vi "GetVersion.vi"() -> ()   [LabVIEW 2013]
uses:
  <vilib>/Platform/fileVersionInfo.llb/FileVersionInformation.ctl
panel:
  out "FileVersionInfo Out":T1
  out "File Version Info":string
  in  "Visible":bool=TRUE
  in  "stop":bool
  in  "Version Message":string
  out "error out":errorcluster
  in  "error in (no error)":errorcluster
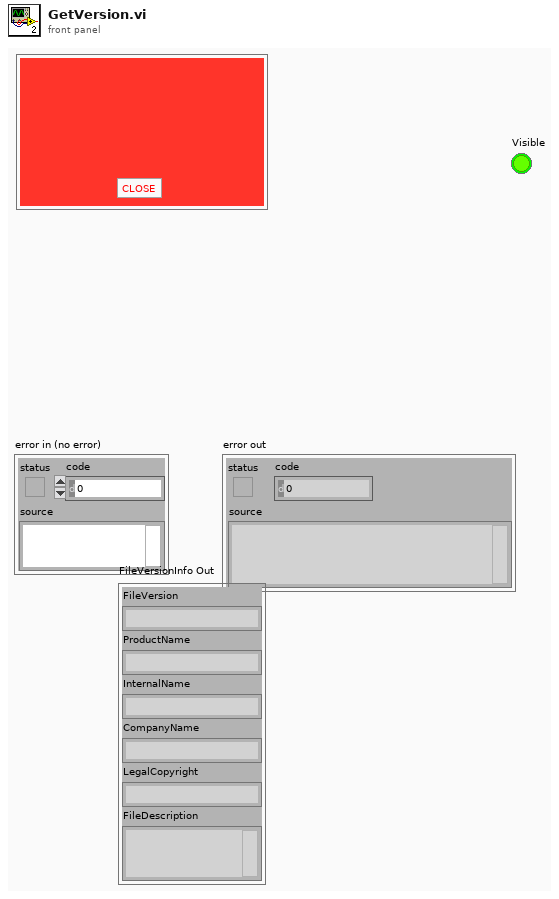
[diagram p1: front panel]
types:
  T1 = typedef "FileVersionInformation.ctl" = cluster{"FileVersion":string, "ProductName":string, "InternalName":string, "CompanyName":string, "LegalCopyright":string, "FileDescription":string}
  T2 = typedef "mysql_authentication.ctl" = cluster{"User":string, "Password":string, "Database":string}
  T3 = cluster{"Port":u16, "IP Address":string, "Authentication":T2}
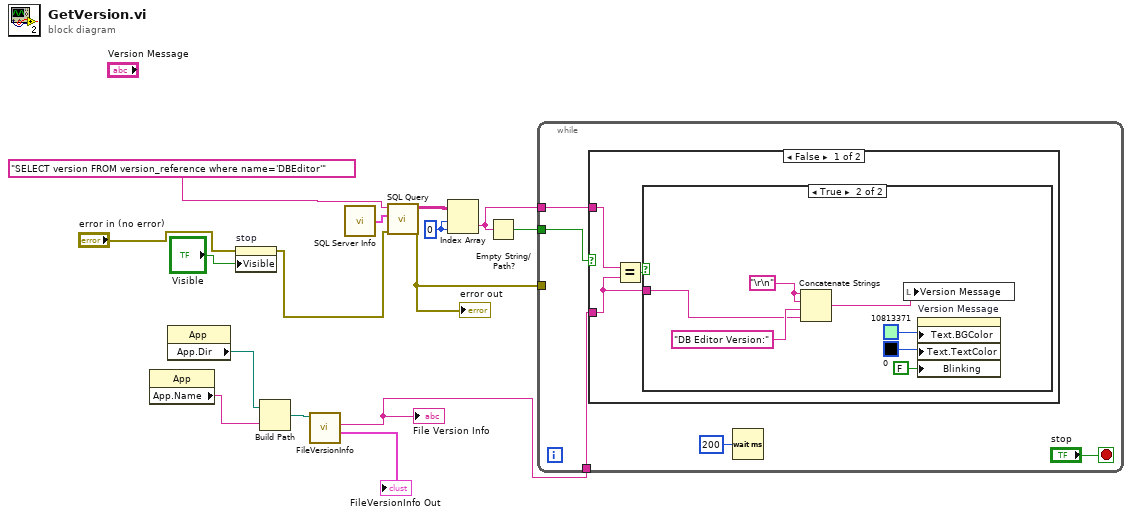
[diagram p0: block diagram]
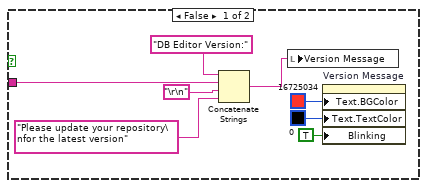
[diagram p2: hidden frame]
diagram:
  w12 = 0 ("disabled index (col)")
  n1 = property class="App"() -> ("App.Name"=w4:string)  [unwired: 2 in, 2 out]
  n2 = property class="App"() -> ("App.Dir"=w5:path)  [unwired: 2 in, 2 out]
  n3 = property on="stop" class="Bool"(error in="error in (no error)", "Visible"="Visible") -> (error out=w7:errorcluster)  [unwired: 1 in, 1 out]
  n4 = Build Path(base path=w5, name or relative path=w4) -> (appended path=w3:path)
  n5 = call <vilib>:"FileVersionInfo.vi"("Application Path in"=w3) -> ("FileVersionInfo Out"=→"FileVersionInfo Out":T1, "File Version Info"=w1:string)  [unwired: 7 in, 2 out]
  "File Version Info" <- w1
  n6 = call "SQL Server Info.vi"() -> ("SQL Server Info"=w14:T3)
  n7 = call "SQL Query.vi"("error in (no error)"=w7, "SQL Server Info"=w14, "Query"="SELECT version FROM version_reference where name='DBEditor'") -> ("error out"=w6:errorcluster, "data"=w15:string[][])  [unwired: 7 in]
  "error out" <- w6
  n8 = Index Array(array=w15, index (row)=w12, index (col)=w12) -> (element=w10:string)
  n9 = Empty String/Path?(string/path=w10) -> (empty?=w11:bool)
  n10 = while {
    tunnel: w11 -> [w20]
    tunnel: w10 -> [w19]
    tunnel: w1 -> [w18]
    tunnel: w6 -> [_]
    stop <- "stop" stop-if-true
    n11 = case shown="False" w20 {
      tunnel: w19 -> [w23 _]
      tunnel: w18 -> [w22 _]
      frame False {
        n12 = Equal?(x=w23, y=w22) -> (x = y?=w21:bool)
        n13 = case shown="True" w21 {
          tunnel: w22 -> [w26 w37]
          frame False {
            n14 = Concatenate Strings("DB Editor Version:" ("Version Message"), w26, "\r\n", "Please update your repository\nfor the latest version" ("string")) -> (w31:string)
            n15 = local write "Version Message"(w31) -> ()
            n16 = property on="Version Message" class="Str"("Text.BGColor"=u32 16725034, "Text.TextColor"=u32 0, "Blinking"=TRUE) -> ()  [unwired: 2 in, 2 out]
          }
          frame True {
            w32 = "\r\n"
            n17 = Concatenate Strings(w32, w32, "DB Editor Version:" ("Version Message"), w37) -> (w36:string)
            n18 = local write "Version Message"(w36) -> ()
            n19 = property on="Version Message" class="Str"("Text.BGColor"=u32 10813371, "Text.TextColor"=u32 0, "Blinking"=FALSE) -> ()  [unwired: 2 in, 2 out]
          }
        }
      }
      frame True {
      }
    }
    n20 = Wait (ms)(milliseconds to wait=u32 200) -> ()  [unwired: 1 out]
  }
